vi "ComputeRotationAndLength.vi"(8 "Y2":dbl format="%#_11g", 9 "X2":dbl format="%#_10g", 10 "Y1":dbl format="%#_11g", 11 "X1":dbl format="%#_11g") -> (3 "Theta (Rad)":dbl format="%#_8g")   [LabVIEW 2018]
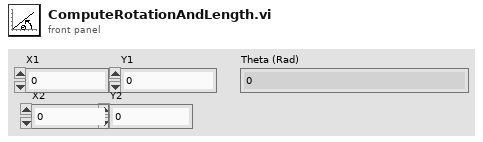
[diagram p1: front panel]
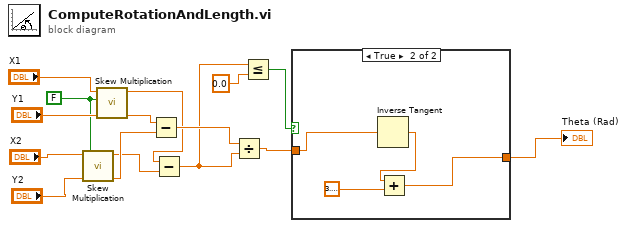
[diagram p0: block diagram]
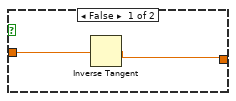
[diagram p2: hidden frame]
diagram:
  w3 = FALSE ("Boolean")
  n1 = call "Skew Multiplication.vi"("Y"="Y2", "Boolean"=w3, "X"="X2") -> ("Y'"=w2:dbl, "X'"=w1:dbl)  [unwired: 7 in]
  n2 = call "Skew Multiplication.vi"("Y"="Y1", "Boolean"=w3, "X"="X1") -> ("Y'"=w6:dbl, "X'"=w8:dbl)  [unwired: 7 in]
  n3 = Subtract(x=w6, y=w2) -> (x-y=w15:dbl)
  n4 = Subtract(x=w8, y=w1) -> (x-y=w14:dbl)
  n5 = Divide(x=w15, y=w14) -> (x/y=w11:dbl)
  n6 = Less Or Equal?(x=w14, y=0.0) -> (x <= y?=w12:bool)
  n7 = case shown="True" w12 {
    tunnel: w11 -> [w17 w20]
    tunnel: [w16 w18] -> w10
    frame False {
      n8 = Inverse Tangent(1:w17) -> (0:w16:dbl)
    }
    frame True {
      n9 = Inverse Tangent(1:w20) -> (0:w21:dbl)
      n10 = Add(x=w21, y=3.141592653589793) -> (x+y=w18:dbl)
    }
  }
  "Theta (Rad)" <- w10
